vi "Get SMO Name from Error Event.vi"(8 "error in (no error)":errorcluster, 9 "Error":refnum<user-event>, 10 "SMOs":refnum<class "SMO.lvclass">[](array[class]), 11 "Logger.Error":refnum<class "Logger.Error.lvclass">) -> (0 "error out":errorcluster, 2 "class:SMO name":string, 3 "Logger.Error out":refnum<class "Logger.Error.lvclass">)   [LabVIEW 2019, in "Logger.Error.lvlib" / "Logger.Error.lvclass"]
uses:
  Logger.Error.lvclass
  <vilib>/JKI/JKI SMO/smo.lvlibp/SMO/SMO.lvclass
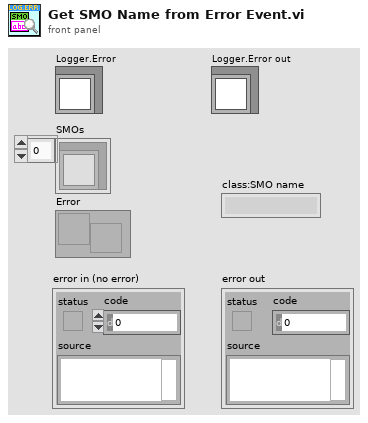
[diagram p1: front panel]
types:
  T1 = typedef "smo.lvlibp/SMO.lvclass/Public Events.ctl" = cluster{"Error":refnum<user-event>, "State":refnum<user-event>, "Reserve State":refnum<user-event>}
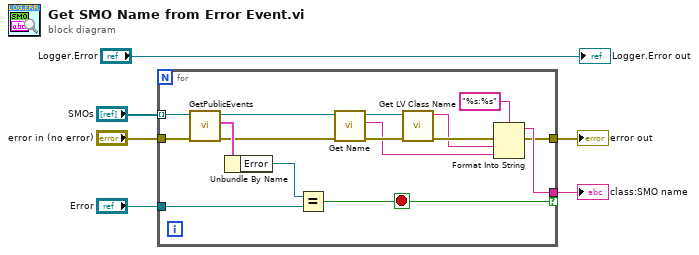
[diagram p0: block diagram]
diagram:
  n1 = for {
    tunnel: "SMOs" -> [w22] mode=indexing
    tunnel: "Error" -> [w19]
    tunnel: [w14] -> w2 if=w15
    tunnel: "error in (no error)" -> [w16]
    tunnel: [w12] -> w3
    stop <- w15 stop-if-true
    n2 = call <vilib>:"GetPublicEvents.vi"("error in (no error)"=w16, "SMO"=w22) -> ("error out"=w9:errorcluster, "Public Events"=w21:T1, "SMO out"=w8:refnum<class "SMO.lvclass">)  [unwired: 7 in]
    n3 = Unbundle By Name(w21) -> ("Error"=w20:refnum<user-event>)
    n4 = Equal?(x=w20, y=w19) -> (x = y?=w15:bool)
    n5 = call <vilib>:"Get Name.vi"("error in (no error)"=w9, "SMO"=w8) -> ("error out"=w17:errorcluster, "Name"=w10:string, "SMO out"=w18:refnum<class "SMO.lvclass">)  [unwired: 5 in, 2 out]
    n6 = call <vilib>:"Get LV Class Name.vi"("error in (no error)"=w17, "object"=w18) -> ("error out"=w13:errorcluster, "class name"=w7:string)  [unwired: 8 in]
    n7 = Format Into String(format string="%s:%s", error in=w13, w7, w10) -> (resulting string=w14:string, error out=w12:errorcluster)  [unwired: 1 in]
  }
  "error out" <- w3
  "class:SMO name" <- w2
  "Logger.Error out" <- "Logger.Error"
